vi "change_plot_units.vi"(7 "PES Display Reference":refnum<vi>, 13 "Controls":T1) -> ()   [LabVIEW 2023]
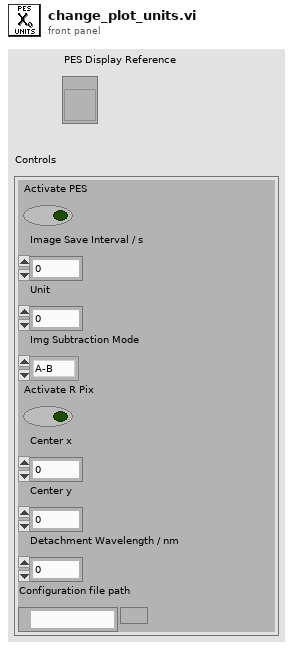
[diagram p1: front panel]
types:
  T1 = cluster{"Activate PES":bool, "Image Save Interval / s":dbl, "Unit":u16, "Img Subtraction Mode":enum16{"A-B", "B-A", "A+B"}, "Activate R Pix":bool, "Center x":i32, "Center y":i32, "Detachment Wavelength / nm":dbl, "Configuration file path":path}
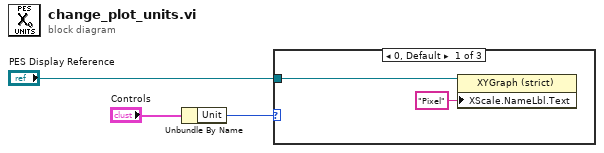
[diagram p0: block diagram]
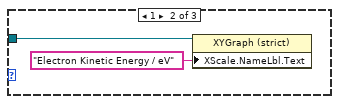
[diagram p2: hidden frame]
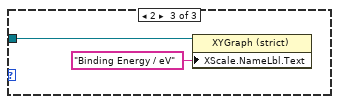
[diagram p3: hidden frame]
diagram:
  n1 = Unbundle By Name("Controls") -> ("Unit"=w2:u16)
  n2 = case shown="0, Default" w2 {
    tunnel: "PES Display Reference" -> [w5 w7 w9]
    frame 0, Default {
      n3 = property class="XYGraph (strict)"(reference=w5, "XScale.NameLbl.Text"="Pixel" ("X Scale.Unit Label.Text")) -> ()  [unwired: 1 in, 2 out]
    }
    frame 1 {
      n4 = property class="XYGraph (strict)"(reference=w7, "XScale.NameLbl.Text"="Electron Kinetic Energy / eV" ("X Scale.Unit Label.Text")) -> ()  [unwired: 1 in, 2 out]
    }
    frame 2 {
      n5 = property class="XYGraph (strict)"(reference=w9, "XScale.NameLbl.Text"="Binding Energy / eV" ("X Scale.Unit Label.Text")) -> ()  [unwired: 1 in, 2 out]
    }
  }
